vi "Set Generation Mode.vi"(8 "error in (no error)":errorcluster, 10 "Mode":T1, 11 "IED in":refnum<class "IED.lvclass">) -> (0 "error out":errorcluster, 3 "IED out":refnum<class "IED.lvclass">)   [LabVIEW 2015, in "IED Actor.lvlib" / "IED.lvclass"]
uses:
  IED.lvclass
  Controls/Generation Mode.ctl
  IED.lvclass/IED.ctl
  <vilib>/NI/Tools/Keyed Array/Map String.vi
  <vilib>/NI/Tools/String/Get Case Matching.vi
  <vilib>/Modbus/master/Modbus Master.lvclass
  <vilib>/NI/Tools/Keyed Array/Tools_KeyedArray.lvlib
  Utilities/Message Strings.llb/Message String Utilities.lvlib
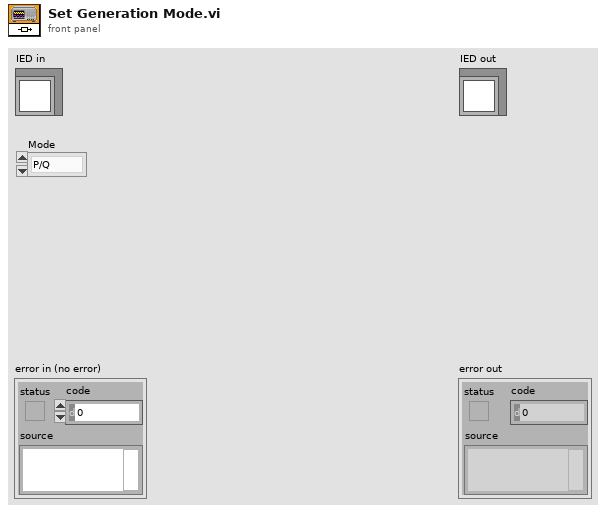
[diagram p1: front panel]
types:
  T1 = typedef "IED Actor.lvlib/IED.lvclass/Generation Mode.ctl" = enum16{"P/Q", "V/f"}
  T2 = typedef "Tools_KeyedArray.lvlib/KeyedArray.ctl" = cluster{"keys":string[], "values":string[]}
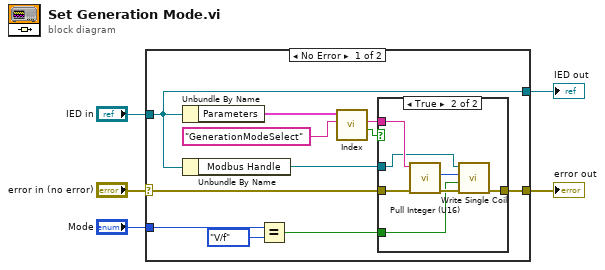
[diagram p0: block diagram]
diagram:
  n1 = case shown="No Error" "error in (no error)" {
    selector: "error in (no error)" -> [w7 w26]
    tunnel: [w6 w26] -> w3
    tunnel: [w12 w25] -> w4
    tunnel: "IED in" -> [w12 w25]
    tunnel: "Mode" -> [w11 _]
    frame No Error {
      n2 = Unbundle By Name(w12) -> ("Parameters"=w16:T2)
      n3 = Unbundle By Name(w12) -> ("Modbus Handle"=w8:refnum<class "Modbus Master.lvclass">)
      n4 = Equal?(x=w11, y=Generation_Mode."V/f") -> (x = y?=w9:bool)
      n5 = call <vilib>:"Index.vi"("key"="GenerationModeSelect", "array in"=w16) -> ("valid key"=w14:bool, "value"=w13:string)  [unwired: 3 in, 1 out]
      n6 = case shown="True" w14 {
        tunnel: w13 -> [_ w24]
        tunnel: w7 -> [w17 w23]
        tunnel: [w17 w20] -> w6
        tunnel: w8 -> [_ w19]
        tunnel: w9 -> [_ w18]
        frame False {
        }
        frame True {
          n7 = call "Pull Integer (U16).vi"("error in (no error)"=w23, "String in"=w24) -> ("error out"=w22:errorcluster, "Integer out"=w21:u16)  [unwired: 7 in, 1 out]
          n8 = call-dynamic "Write Single Coil.vi"("error in (no error)"=w22, "coil value"=w18, "address"=w21, "Modbus master in"=w19) -> ("error out"=w20:errorcluster)  [unwired: 6 in, 1 out]
        }
      }
    }
    frame Error {
    }
  }
  "error out" <- w3
  "IED out" <- w4
